vi "Do.vi"(8 "Error In":errorcluster, 10 "Actor In":refnum<class "Actor.lvclass">, 11 "Register Msg":refnum<class "Register Msg.lvclass">) -> (0 "Error Out":errorcluster, 2 "Actor Out":refnum<class "Actor.lvclass">)   [LabVIEW 2015, in "Event Source.lvlib" / "Register Msg.lvclass"]
doc: "This VI delivers the message to the actor by calling the appropriate method(s) on the actor."
uses:
  Register Msg.lvclass
  Event Source/Event Source.lvclass
  <vilib>/ActorFramework/Actor/Actor.lvclass
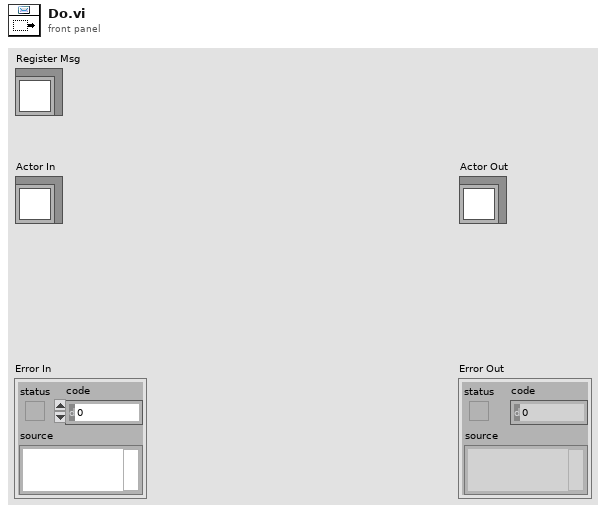
[diagram p1: front panel]
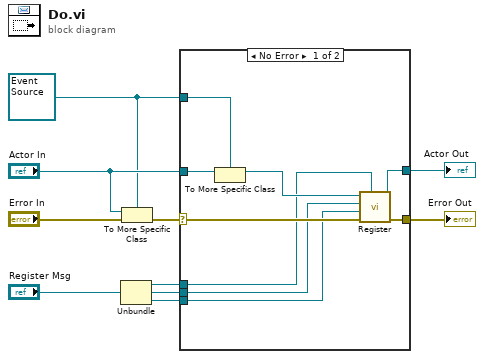
[diagram p0: block diagram]
diagram:
  w4 = refnum<class "Event Source.lvclass"> refnum ("Actor in")
  n1 = Unbundle("Register Msg") -> (w3:refnum<class "Event.lvclass">, w2:refnum<class "Message Enqueuer.lvclass">, w1:refnum<class "Event Generated Msg.lvclass">)
  n2 = To More Specific Class(target class=w4, reference="Actor In", error in="Error In") -> (error out=w8:errorcluster)  [unwired: 1 out]
  n3 = case shown="No Error" w8 {
    selector: w8 -> [w17 w21]
    tunnel: [w19 w21] -> w7
    tunnel: [w18 w20] -> w6
    tunnel: "Actor In" -> [w16 w20]
    tunnel: w4 -> [w15 _]
    tunnel: w3 -> [w13 _]
    tunnel: w2 -> [w12 _]
    tunnel: w1 -> [w11 _]
    frame No Error {
      n4 = To More Specific Class(target class=w15, reference=w16) -> (specific class reference=w14:refnum<class "Event Source.lvclass">)  [unwired: 1 in, 1 out]
      n5 = call "Register.vi"("Event"=w13, "Error In"=w17, "Event Fire Handler"=w11, "Registrant Enq"=w12, "Event Source In"=w14) -> ("Error Out"=w19:errorcluster, "Event Source Out"=w18:refnum<class "Event Source.lvclass">)  [unwired: 5 in]
    }
    frame Error {
      # "If type check fails, pass the original object out again."
    }
  }
  "Error Out" <- w7
  "Actor Out" <- w6
